vi "Draw Shading for Range Cursors.vi"(10 "WaveformGraph":refnum<vi>, 11 "Display State In":T1={"Graph Visible Items"={"Plot Legend"=FALSE, "Scale Legend"=FALSE, "Graph Palette"=FALSE, "Cursor Legend"=FALSE, "X Scrollbar"=FALSE}, "View Table"=FALSE, "Table Visible Items"={"Vertical Scrollbar"=FALSE, "Horizontal Scrollbar"=FALSE, "Row Headers"=FALSE, "Column Headers"=FALSE, "Vertical Lines"=FALSE, "Horizontal Lines"=FALSE}, "Header Font"={"Font Name"="", "Size"=0, "Bold"=FALSE, "Italic"=FALSE, "Underline"=FALSE, "Strikeout"=FALSE, "Color"=0}, "Cell Font"={"Font Name"="", "Size"=0, "Bold"=FALSE, "Italic"=FALSE, "Underline"=FALSE, "Strikeout"=FALSE, "Color"=0}, "Description and Tip..."={"Description"="", "Tip"=""}, "Moveable Splitter Position"=0, "Measurement Cursor Configuration"={"relative to t0"={"enable relative time"=FALSE, "Relative times (DT)"=[], "color"=0}, "range"={"enable range"=FALSE, "T1"=0.0, "T2"=0.0, "Fixed interval (T2-T1)"=0.0, "T1 color"=0, "T2 color"=0, "enable shading"=FALSE}, "periodic"={"enable periodic"=FALSE, "First event (E1)"=0.0, "Number events (Ei)"=0, "Event spacing (s)"=0.0, "First color"=0, "Events color"=0}, "absolute timestamp"={"enable absolute"=FALSE, "Timestamps (TS)"=[], "color"=0}}, "X Increment"=0.0, "X Scale"={"Label Visible"=FALSE, "Label Text"="", "Time Mode"=enum."Relative", "Format String"=""}, "Y Scale"={"Label Visible"=FALSE, "Label Text"="", "Scaling"=enum."Engineering Units", "Format String"=""}, "Colors"={"background"=16777215, "major grid"=8355711, "minor grid"=12632256, "font"=0}, "Cursors"={"List"=[], "Tags"=[]}, "Plots"=[], "Plot Color Wheel"=[3381759, 32768, 982784, 4375295, 13827953, 13457919, 16757522, 4343295, 16728758, 12095254], "registered user events"=variant} caption="State") -> (3 "Display State Out":T1={"Graph Visible Items"={"Plot Legend"=FALSE, "Scale Legend"=FALSE, "Graph Palette"=FALSE, "Cursor Legend"=FALSE, "X Scrollbar"=FALSE}, "View Table"=FALSE, "Table Visible Items"={"Vertical Scrollbar"=FALSE, "Horizontal Scrollbar"=FALSE, "Row Headers"=FALSE, "Column Headers"=FALSE, "Vertical Lines"=FALSE, "Horizontal Lines"=FALSE}, "Header Font"={"Font Name"="", "Size"=0, "Bold"=FALSE, "Italic"=FALSE, "Underline"=FALSE, "Strikeout"=FALSE, "Color"=0}, "Cell Font"={"Font Name"="", "Size"=0, "Bold"=FALSE, "Italic"=FALSE, "Underline"=FALSE, "Strikeout"=FALSE, "Color"=0}, "Description and Tip..."={"Description"="", "Tip"=""}, "Moveable Splitter Position"=0, "Measurement Cursor Configuration"={"relative to t0"={"enable relative time"=FALSE, "Relative times (DT)"=[], "color"=0}, "range"={"enable range"=FALSE, "T1"=0.0, "T2"=0.0, "Fixed interval (T2-T1)"=0.0, "T1 color"=0, "T2 color"=0, "enable shading"=FALSE}, "periodic"={"enable periodic"=FALSE, "First event (E1)"=0.0, "Number events (Ei)"=0, "Event spacing (s)"=0.0, "First color"=0, "Events color"=0}, "absolute timestamp"={"enable absolute"=FALSE, "Timestamps (TS)"=[], "color"=0}}, "X Increment"=0.0, "X Scale"={"Label Visible"=FALSE, "Label Text"="", "Time Mode"=enum."Relative", "Format String"=""}, "Y Scale"={"Label Visible"=FALSE, "Label Text"="", "Scaling"=enum."Engineering Units", "Format String"=""}, "Colors"={"background"=16777215, "major grid"=8355711, "minor grid"=12632256, "font"=0}, "Cursors"={"List"=[], "Tags"=[]}, "Plots"=[], "Plot Color Wheel"=[3381759, 32768, 982784, 4375295, 13827953, 13457919, 16757522, 4343295, 16728758, 12095254], "registered user events"=variant} caption="State")   [LabVIEW 2017, in "Waveforms with Cursors.xctl"]
uses:
  <vilib>/addons/_XControls/Waveforms with Cursors/Waveforms with Cursors.xctl
  <vilib>/addons/_XControls/Waveforms with Cursors/Controls/State.ctl
  <vilib>/Utility/miscctls.llb/LVFontTypeDef.ctl
  <vilib>/addons/_XControls/Waveforms with Cursors/Controls/Waveform Cursor Configuration.ctl
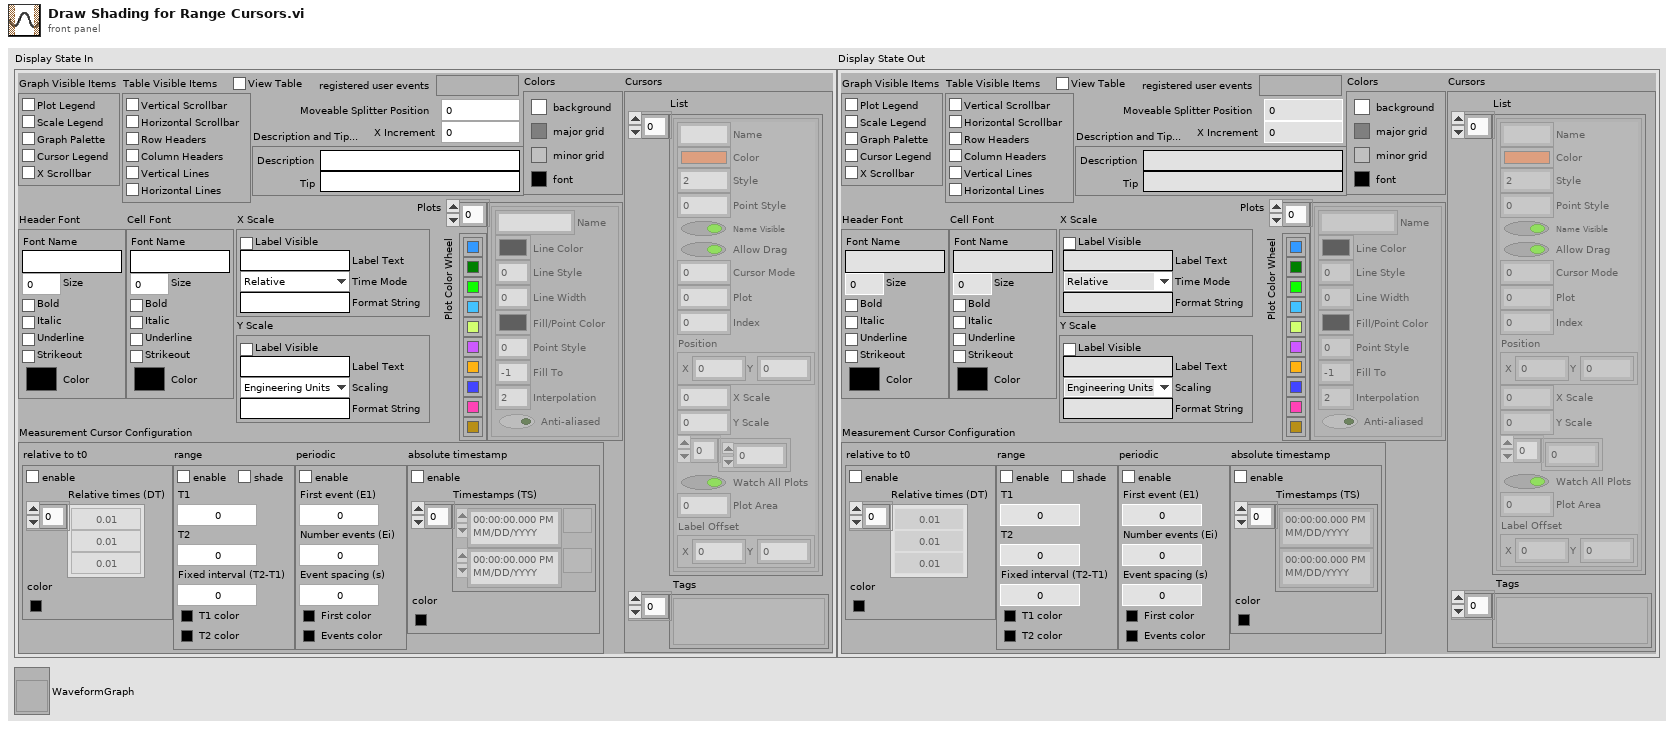
[diagram p1: front panel]
types:
  T1 = typedef "Waveforms with Cursors.xctl/State.ctl" = cluster{"Graph Visible Items":cluster{"Plot Legend":bool, "Scale Legend":bool, "Graph Palette":bool, "Cursor Legend":bool, "X Scrollbar":bool}, "View Table":bool, "Table Visible Items":cluster{"Vertical Scrollbar":bool, "Horizontal Scrollbar":bool, "Row Headers":bool, "Column Headers":bool, "Vertical Lines":bool, "Horizontal Lines":bool}, "Header Font":T2, "Cell Font":T2, "Description and Tip...":cluster{"Description":string, "Tip":string}, "Moveable Splitter Position":i32, "Measurement Cursor Configuration":T3, "X Increment":dbl, "X Scale":cluster{"Label Visible":bool, "Label Text":string, "Time Mode":enum16{"Relative", "Absolute"}, "Format String":string}, "Y Scale":cluster{"Label Visible":bool, "Label Text":string, "Scaling":enum16{"Engineering Units", "Voltage"}, "Format String":string}, "Colors":cluster{"background":u32, "major grid":u32, "minor grid":u32, "font":u32}, "Cursors":cluster{"List":cluster{"Name":string, "Color":u32, "Style":i32, "Point Style":u8, "Name Visible":bool, "Allow Drag":bool, "Cursor Mode":u32, "Plot":i32, "Index":i32, "Position":cluster{"X":dbl, "Y":dbl}, "X Scale":u32, "Y Scale":u32, "Watch Plots":i32[], "Watch All Plots":bool, "Plot Area":i32, "Label Offset":cluster{"X":dbl, "Y":dbl}}[], "Tags":variant[]}, "Plots":cluster{"Name":string, "Line Color":u32, "Line Style":u8, "Line Width":u8, "Fill/Point Color":u32, "Point Style":u8, "Fill To":i16, "Interpolation":u8, "Anti-aliased":bool}[], "Plot Color Wheel":u32[], "registered user events":variant}
  T2 = typedef "LVFontTypeDef.ctl" = cluster{"Font Name":string, "Size":u16, "Bold":bool, "Italic":bool, "Underline":bool, "Strikeout":bool, "Color":u32}
  T3 = typedef "Waveforms with Cursors.xctl/Waveform Cursor Configuration.ctl" = cluster{"relative to t0":cluster{"enable relative time":bool, "Relative times (DT)":dbl[], "color":u32}, "range":cluster{"enable range":bool, "T1":dbl, "T2":dbl, "Fixed interval (T2-T1)":dbl, "T1 color":u32, "T2 color":u32, "enable shading":bool}, "periodic":cluster{"enable periodic":bool, "First event (E1)":dbl, "Number events (Ei)":i32, "Event spacing (s)":dbl, "First color":u32, "Events color":u32}, "absolute timestamp":cluster{"enable absolute":bool, "Timestamps (TS)":timestamp[], "color":u32}}
  T4 = cluster{"left":i16, "top":i16, "right":i16, "bottom":i16}
  T5 = typedef "LVRectTypeDef.ctl" = cluster{"Left":i16, "Top":i16, "Right":i16, "Bottom":i16}
  T6 = typedef "LVPoint32TypeDef.ctl" = cluster{"Horizontal":i32, "Vertical":i32}
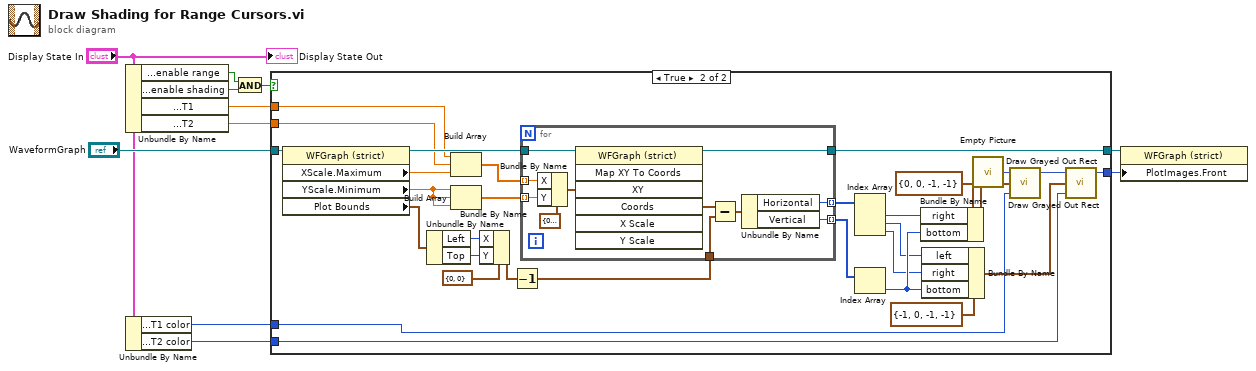
[diagram p0: block diagram]
diagram:
  n1 = Unbundle By Name("Display State In") -> ("Measurement Cursor Configuration.range.enable range"=w3:bool, "Measurement Cursor Configuration.range.enable shading"=w2:bool, "Measurement Cursor Configuration.range.T1"=w10:dbl, "Measurement Cursor Configuration.range.T2"=w9:dbl)
  n2 = Unbundle By Name("Display State In") -> ("Measurement Cursor Configuration.range.T1 color"=w7:u32, "Measurement Cursor Configuration.range.T2 color"=w6:u32)
  n3 = And(x=w3, y=w2) -> (x .and. y?=w1:bool)
  n4 = case shown="True" w1 {
    tunnel: "WaveformGraph" -> [w12 w37]
    tunnel: w10 -> [_ w18]
    tunnel: w9 -> [_ w17]
    tunnel: w7 -> [_ w16]
    tunnel: w6 -> [_ w15]
    tunnel: [_ w14] -> w5
    tunnel: [w12 w13] -> w4
    frame False {
    }
    frame True {
      n5 = property class="WFGraph (strict)"(reference=w37) -> (reference out=w42:refnum<vi>, "XScale.Maximum"=w38:dbl, "YScale.Minimum"=w39:dbl, "Plot Bounds"=w40:T5)  [unwired: 1 in, 1 out]
      n6 = Unbundle By Name(w40) -> ("Left"=w21:i16, "Top"=w22:i16)
      n7 = Build Array(w18, w17, w38) -> (w19:dbl[])
      n8 = Build Array(w39, w39, w39) -> (w20:dbl[])
      n9 = Bundle By Name(cluster=cluster{"X":i16, "Y":i16} {"X"=0, "Y"=0} ("XY"), "X"=w21, "Y"=w22) -> (w23:cluster{"X":i16, "Y":i16})
      n10 = Decrement(x=w23) -> (x-1=w41:cluster{"X":i16, "Y":i16})
      n11 = for {
        tunnel: w19 -> [w53] mode=indexing
        tunnel: w20 -> [w52] mode=indexing
        tunnel: [w50] -> w31 mode=indexing
        tunnel: [w49] -> w32 mode=indexing
        tunnel: w41 -> [w47]
        tunnel: w42 -> [w44]
        tunnel: [w43] -> w13
        n12 = Bundle By Name(cluster=cluster{"X":dbl, "Y":dbl} {"X"=0.0, "Y"=0.0} ("XY"), "X"=w53, "Y"=w52) -> (w46:cluster{"X":dbl, "Y":dbl})
        n13 = invoke class="WFGraph (strict)" method="Map XY To Coords"(reference=w44, "XY"=w46) -> (reference out=w43:refnum<vi>, "Coords"=w45:T6)  [unwired: 5 in, 5 out]
        n14 = Subtract(x=w45, y=w47) -> (x-y=w51:T6)
        n15 = Unbundle By Name(w51) -> ("Horizontal"=w50:i32, "Vertical"=w49:i32)
      }
      n16 = Index Array(array=w31) -> (element #1=w33:i32, element #2=w34:i32, element #3=w35:i32)  [unwired: 3 in]
      n17 = Index Array(array=w32) -> (element=w36:i32)  [unwired: 1 in]
      n18 = Bundle By Name(cluster=T4 {"left"=0, "top"=0, "right"=-1, "bottom"=-1} ("rect"), "right"=w33, "bottom"=w36) -> (w28:T4)
      n19 = Bundle By Name(cluster=T4 {"left"=-1, "top"=0, "right"=-1, "bottom"=-1} ("rect"), "left"=w34, "right"=w35, "bottom"=w36) -> (w30:T4)
      n20 = call "Empty Picture"() -> ("empty picture"=w27:picture)
      n21 = call <vilib>:"Draw Grayed Out Rect.vi"("color(black)"=w16, "rect"=w28, "picture"=w27) -> ("new picture"=w29:picture)  [unwired: 2 in]
      n22 = call <vilib>:"Draw Grayed Out Rect.vi"("color(black)"=w15, "rect"=w30, "picture"=w29) -> ("new picture"=w14:picture)  [unwired: 2 in]
    }
  }
  n23 = property class="WFGraph (strict)"(reference=w4, "PlotImages.Front"=w5) -> ()  [unwired: 1 in, 2 out]
  "Display State Out" <- "Display State In"
